vi "Stream References.vi"() -> ()   [LabVIEW 2014]
panel:
  out "RT Writer":refnum<k21>
  out "RT Reader":refnum<k21>
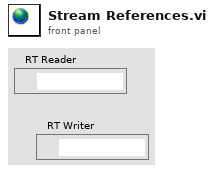
[diagram p1: front panel]
diagram:
